vi "LVClass_HasoSlopes ctor from Image.vi"(0 "HasoSlopes in":refnum<class "HasoSlopes.lvclass">, 5 "Image.lvclass":refnum<class "Image.lvclass">, 7 "Haso configuration file":path, 9 "start subpupil":T1, 11 "error in (no error)":errorcluster) -> (4 "HasoSlopes out":refnum<class "HasoSlopes.lvclass">, 15 "error out":errorcluster)   [LabVIEW 2020, in "HasoSlopes.lvclass"]
uses:
  HasoSlopes.lvclass
  Image.lvclass
  Point2D.ctl
  Handle creation.ctl
  HasoSlopes.lvclass/HasoSlopes.ctl
  LVClass_Image Read Image.vi
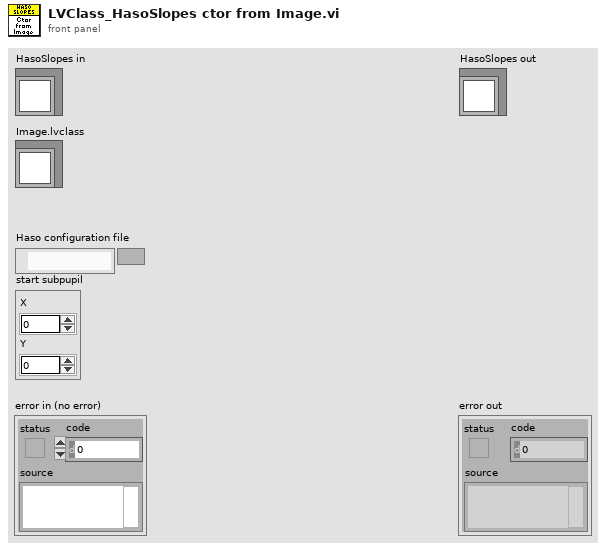
[diagram p1: front panel]
types:
  T1 = typedef "Point2D.ctl" = cluster{"X":u32, "Y":u32}
  T2 = typedef "Handle creation.ctl" = enum16{"By ctor", "By write function"}
  T3 = typedef "Struct_Image.ctl" = cluster{"Image_Handler":i32, "Number of bits":T4, "ImageSize":T1}
  T4 = typedef "Data alignment enum.ctl" = enum16{"8", "16", "32"}
  T5 = typedef "HasoSpecifications.ctl" = cluster{"Serial number":string, "Revision":string, "Model":string, "Dimensions_um":T6, "Pixel position for alignment":T7, "Radius tolerance":u16, "Default start subaperture_sspp":T1, "Lower calibration wavelength_nm":dbl, "Upper calibration wavelength_nm":dbl, "Black subaperture position_sspp":T1, "TiltLimit_mrad":dbl, "Radius_m":dbl, "Smearing limit wavelength_nm":dbl, "Smearing limit exposure duration_us":dbl, "Focal_um":dbl}
  T6 = typedef "General dimensions definition.ctl" = cluster{"Size":T1, "Step":T7}
  T7 = typedef "Point2Df.ctl" = cluster{"X":sgl, "Y":sgl}
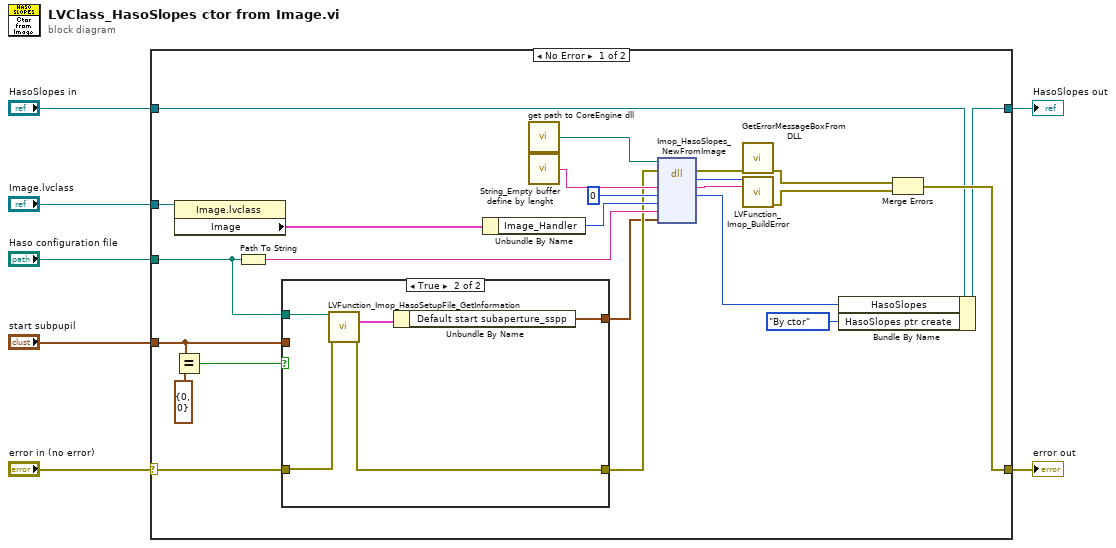
[diagram p0: block diagram]
diagram:
  n1 = case shown="No Error" "error in (no error)" {
    selector: "error in (no error)" -> [w11 w40]
    tunnel: [w24 w40] -> w6
    tunnel: [w22 w39] -> w4
    tunnel: "HasoSlopes in" -> [w23 w39]
    tunnel: "Image.lvclass" -> [w19 _]
    tunnel: "Haso configuration file" -> [w12 _]
    tunnel: "start subpupil" -> [w9 _]
    frame No Error {
      n2 = Equal?(x=w9, y=T1 {"X"=0, "Y"=0}) -> (x = y?=w13:bool)
      n3 = property class="Image.lvclass"(reference=w19) -> ("Image"=w18:T3)  [unwired: 1 in, 2 out]
      n4 = Path To String(path=w12) -> (string=w16:string)
      n5 = case shown="True" w13 {
        tunnel: w12 -> [_ w38]
        tunnel: w11 -> [w32 w36]
        tunnel: [w32 w35] -> w10
        tunnel: [w33 w34] -> w8
        tunnel: w9 -> [w33 _]
        frame False {
        }
        frame True {
          n6 = call "LVFunction_Imop_HasoSetupFile_GetInformation.vi"("module path"=w38, "error in (no error)"=w36) -> ("HASO specifications"=w37:T5, "error out"=w35:errorcluster)  [unwired: 10 in, 2 out]
          n7 = Unbundle By Name(w37) -> ("Default start subaperture_sspp"=w34:T1)
        }
      }
      n8 = Unbundle By Name(w18) -> ("Image_Handler"=w17:i32)
      n9 = call "get path to CoreEngine dll.vi"() -> ("path to c_interface_vc100.dll"=w27:path)  [unwired: 12 in, 3 out]
      n10 = call "String_Empty buffer define by lenght.vi"() -> ("Empty buffer"=w28:string)  [unwired: 1 in]
      n11 = dll-call lib="D:/FLE/0.Code/CoreEngine4_Suite/LV2011_interface/DLLs/c_interface_vc100.dll" fn="Imop_HasoSlopes_NewFromImage"(path in=w27, error in=w10, "Message"=w28, "HasoSlopes"=0, "Image"=w17, "HASO configuration path"=w16, "start subpupil"=w8) -> (error out=w31:errorcluster, "return type"=w29:i32, "Message"=w30:string, "HasoSlopes"=w15:i32)  [unwired: 4 in, 1 out]
      n12 = call "GetErrorMessageBoxFromDLL.vi"("error IN"=w31) -> ("error OUT"=w26:errorcluster)  [unwired: 10 in]
      n13 = call "LVFunction_Imop_BuildError.vi"("code"=w29, "String to Prepend to source (\"\")"=w30) -> ("error out"=w25:errorcluster)  [unwired: 13 in]
      n14 = Bundle By Name(cluster=w23, "HasoSlopes"=w15, "HasoSlopes ptr create"=Handle_creation."By ctor") -> (w22:refnum<class "HasoSlopes.lvclass">)
      n15 = Merge Errors(w26, w25) -> (w24:errorcluster)
    }
    frame Error {
    }
  }
  "error out" <- w6
  "HasoSlopes out" <- w4
